vi "DelArrayEnd.vi"   [LabVIEW 2010]
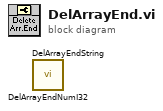
[diagram p0: block diagram]
diagram:
  n1 = call <userlib>:"DelArrayEndNumI32.vi"() -> ()  [unwired: 10 in, 2 out]
  n2 = call <userlib>:"DelArrayEndString.vi"() -> ()  [unwired: 10 in, 2 out]
